vi "Filter_LDA.vi"(8 "Cluster in":T1={"Colour"=0, "Inst type"=enum."Pitot-static tube", "Inst name"="Manometer voltage", "Symbol"="U", "Code name"="", "Extra Info"="U", "Inst Array"=enum."PWA", "Extra Titles"=[], "Extra Values"=[], "Eng Values"=[], "Time (ms)"=[], "Voltage"=[], "U"=0.0, "u^2"=0.0, "u^3"=0.0, "u^4"=0.0, "Skew_u"=0.0, "Kurt_u"=0.0, "Sd Error in Mean"=0.0, "% u'/U"=0.0, "X"=0.0, "Y"=0.0, "Z"=0.0, "Spectra"={"First Name"="", "Second Name"="", "X axis name"="", "Y axis name"="", "X array"=[], "Y array"=[]}, "Autocorrelation"={"First Name"="", "Second Name"="", "X axis name"="", "Y axis name"="", "X array"=[], "Y array"=[]}, "Timescale integral to 25%"=0.0, "Sd Error in Variance"=0.0, "Calib File"=path "", "Calib Constants"=[], "Histogram"={"First Name"="", "Second Name"="", "X axis name"="", "Y axis name"="", "X array"=[], "Y array"=[]}, "Output Position"=FALSE, "Full Stats"=FALSE, "Weighting"=[], "Av Sampling Rate"=0.0, "Av No of Samples"=0.0, "Total Meas Time (s)"=0.0} {"Sd Error in Variance" format="%.2f"; "Skew_u" format="%.2f"; "% u'/U" format="%.2f"; "Sd Error in Mean" format="%.2f"; "Kurt_u" format="%.2f"; "u^4" format="%.2f"; "u^3" format="%.2f"; "U" format="%.2f"; "u^2" format="%.2f"}) -> (3 "Cluster Out":T1={"Colour"=0, "Inst type"=enum."Pitot-static tube", "Inst name"="Manometer voltage", "Symbol"="U", "Code name"="", "Extra Info"="U", "Inst Array"=enum."PWA", "Extra Titles"=[], "Extra Values"=[], "Eng Values"=[], "Time (ms)"=[], "Voltage"=[], "U"=0.0, "u^2"=0.0, "u^3"=0.0, "u^4"=0.0, "Skew_u"=0.0, "Kurt_u"=0.0, "Sd Error in Mean"=0.0, "% u'/U"=0.0, "X"=0.0, "Y"=0.0, "Z"=0.0, "Spectra"={"First Name"="", "Second Name"="", "X axis name"="", "Y axis name"="", "X array"=[], "Y array"=[]}, "Autocorrelation"={"First Name"="", "Second Name"="", "X axis name"="", "Y axis name"="", "X array"=[], "Y array"=[]}, "Timescale integral to 25%"=0.0, "Sd Error in Variance"=0.0, "Calib File"=path "", "Calib Constants"=[], "Histogram"={"First Name"="", "Second Name"="", "X axis name"="", "Y axis name"="", "X array"=[], "Y array"=[]}, "Output Position"=FALSE, "Full Stats"=FALSE, "Weighting"=[], "Av Sampling Rate"=0.0, "Av No of Samples"=0.0, "Total Meas Time (s)"=0.0} {"Sd Error in Variance" format="%.2f"; "Skew_u" format="%.2f"; "% u'/U" format="%.2f"; "Sd Error in Mean" format="%.2f"; "Kurt_u" format="%.2f"; "u^4" format="%.2f"; "u^3" format="%.2f"; "U" format="%.2f"; "u^2" format="%.2f"})   [LabVIEW 2011]
uses:
  Controls/Analysis_info_cluster.ctl
  Controls/Inst_type.ctl
  Controls/Instrument_Array.ctl
  Controls/XY_Plot_Cluster.ctl
  <vilib>/gmath/NI_Gmath.lvlib
panel:
  in  "Cutoff frequency (Hz)":dbl=25.0
  out "Numeric":dbl
  in  "method":i32(ring) items=["nearest", "linear", "spline", "cubic Hermite", "Lagrange"]
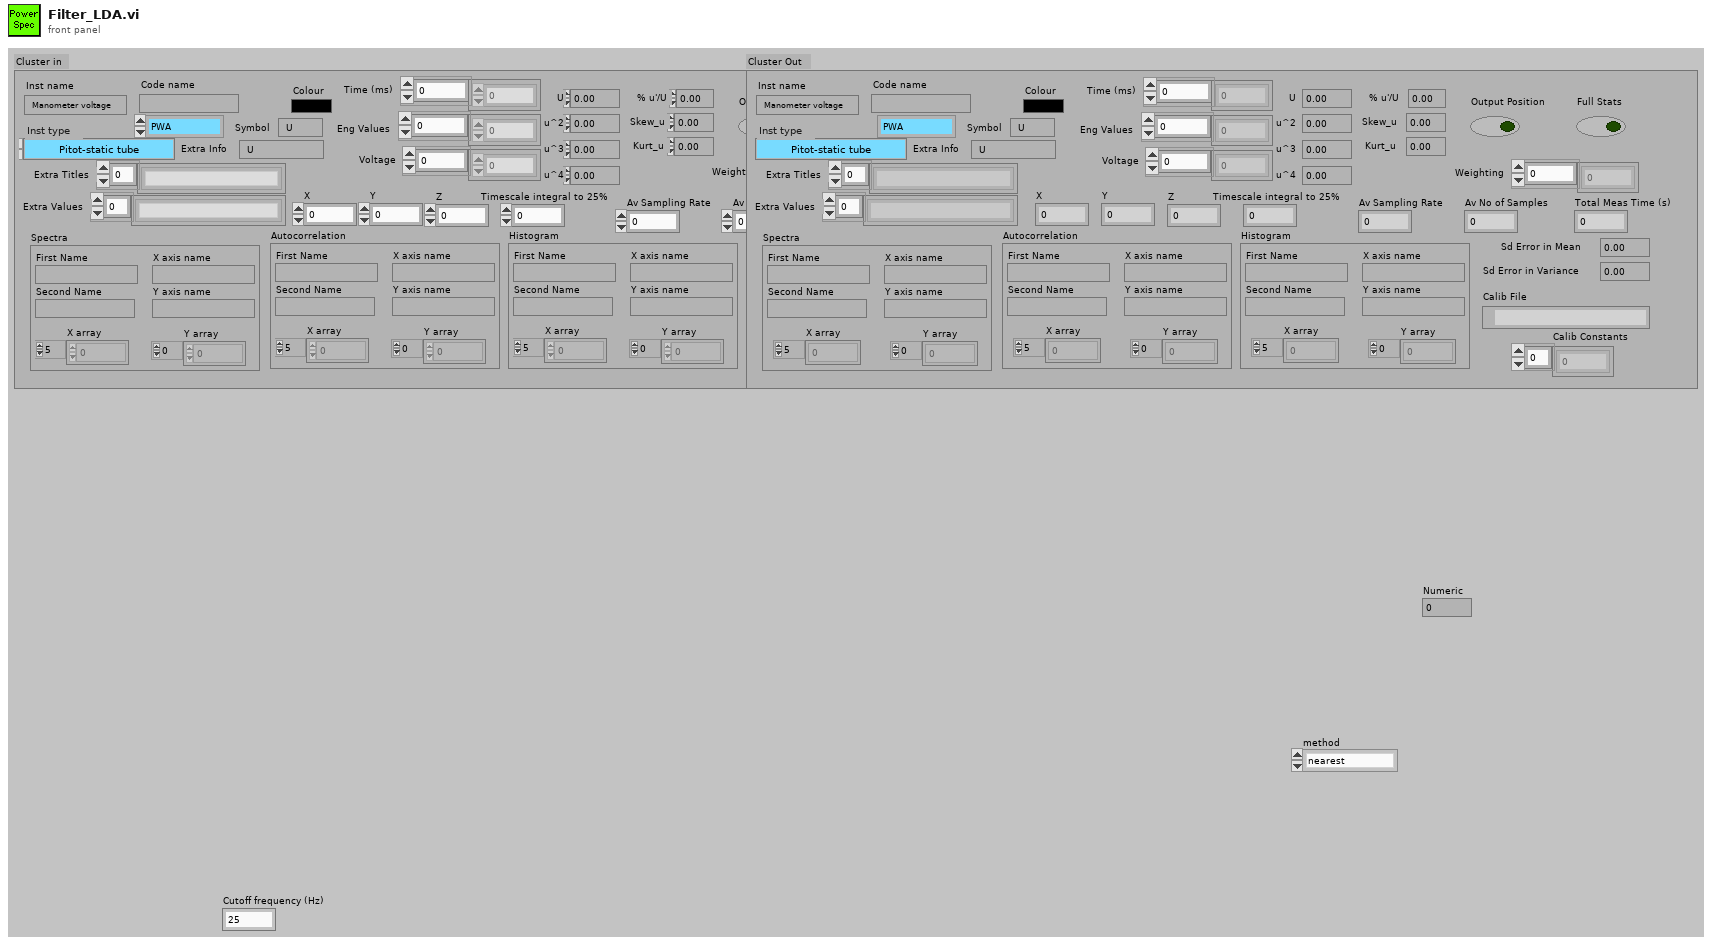
[diagram p1: front panel]
types:
  T1 = typedef "Analysis_info_cluster.ctl" = cluster{"Colour":u32, "Inst type":T2, "Inst name":string, "Symbol":string, "Code name":string, "Extra Info":string, "Inst Array":T3, "Extra Titles":string[], "Extra Values":string[], "Eng Values":dbl[], "Time (ms)":dbl[], "Voltage":dbl[], "U":dbl, "u^2":dbl, "u^3":dbl, "u^4":dbl, "Skew_u":dbl, "Kurt_u":dbl, "Sd Error in Mean":dbl, "% u'/U":dbl, "X":dbl, "Y":dbl, "Z":dbl, "Spectra":T4, "Autocorrelation":T4, "Timescale integral to 25%":dbl, "Sd Error in Variance":dbl, "Calib File":path, "Calib Constants":dbl[], "Histogram":T4, "Output Position":bool, "Full Stats":bool, "Weighting":dbl[], "Av Sampling Rate":dbl, "Av No of Samples":dbl, "Total Meas Time (s)":dbl}
  T2 = typedef "Inst_type.ctl" = enum16{"Propeller anemometer", "Raw voltage", "Pressure Transducer", "Pitot-static tube", "Preston tube", "Hot wire", "Cross wire 1", "Cross wire 2", "Generic Linear", "Generic Polynomial", "Generic BackPoly", "Fast FID", "Thermocouple", "Cold wire", "Pulsed Wire", "LDA Vel", "LDA Tran time", "LDA Arr time"}
  T3 = typedef "Instrument_Array.ctl" = enum16{"PWA", "LDA", "Analogue"}
  T4 = typedef "XY_Plot_Cluster.ctl" = cluster{"First Name":string, "Second Name":string, "X axis name":string, "Y axis name":string, "X array":dbl[], "Y array":dbl[]}
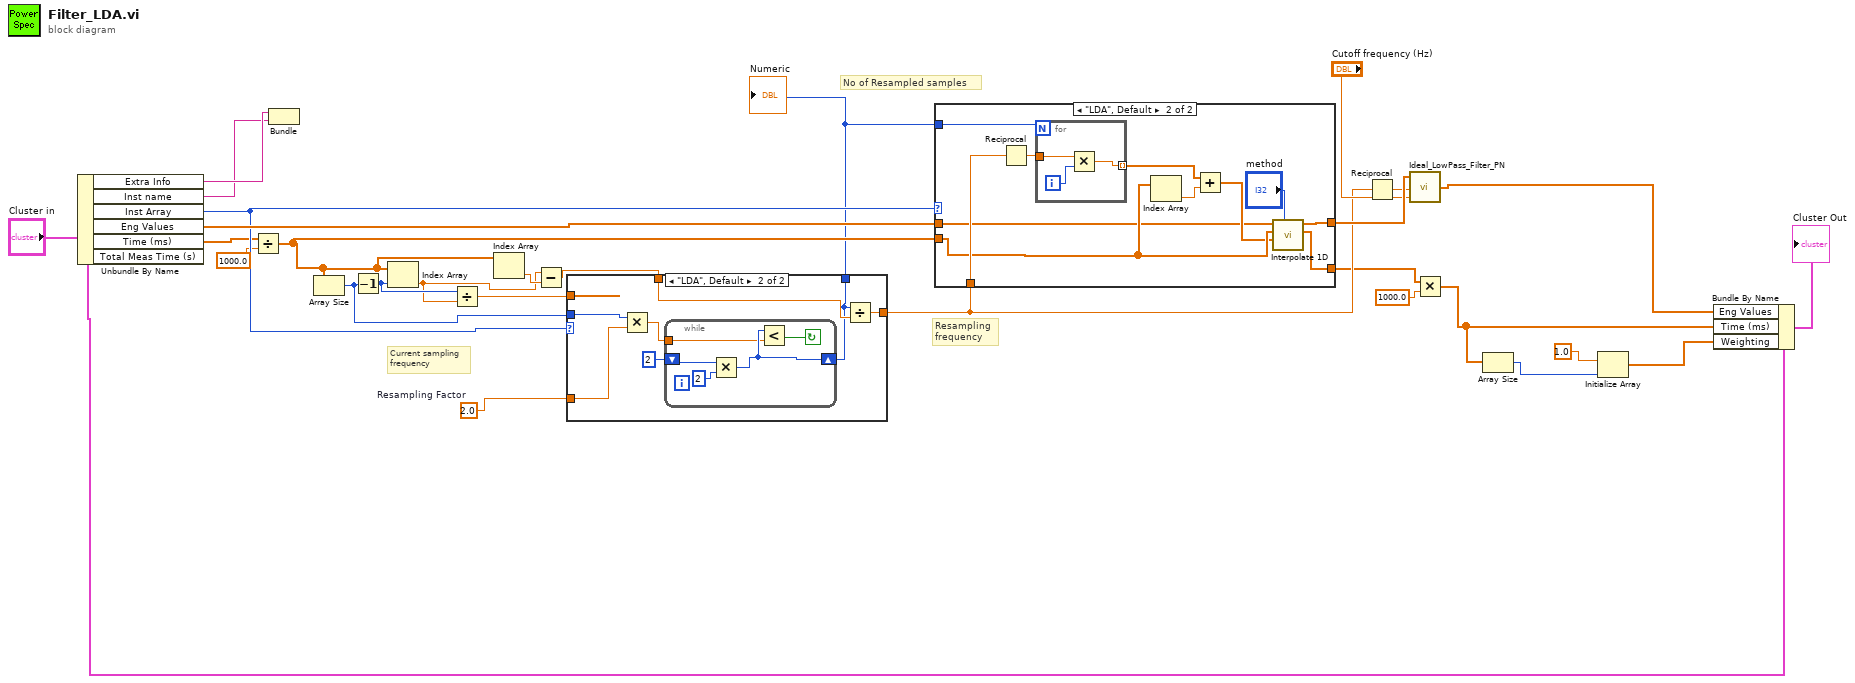
[diagram p0: block diagram]
diagram:
  w7 = 2.0  # Resampling Factor
  # "Current sampling\nfrequency"
  # "No of Resampled samples"
  # "Resampling\nfrequency"
  n1 = Unbundle By Name("Cluster in") -> ("Extra Info"=w23:string, "Inst name"=w22:string, "Inst Array"=w27:T3, "Eng Values"=w28:dbl[], "Time (ms)"=w25:dbl[])  [unwired: 1 out]
  n2 = Divide(x=w25, y=1000.0) -> (x/y=w24:dbl[])
  n3 = Bundle("Extra Info"=w23, "Inst name"=w22) -> ()  [unwired: 1 in, 1 out]
  n4 = Array Size(array=w24) -> (size(s)=w8:i32)
  n5 = Decrement(x=w8) -> (x-1=w9:i32)
  n6 = Index Array(array=w24, index=w9) -> (element=w4:dbl)
  n7 = Divide(x=w9, y=w4) -> (x/y=w10:dbl)
  n8 = Index Array(array=w24) -> (element=w6:dbl)  [unwired: 1 in]
  n9 = Subtract(x=w4, y=w6) -> (x-y=w5:dbl)
  n10 = case shown="\"LDA\", Default" w27 {
    tunnel: w10 -> [w30 _]
    tunnel: w5 -> [_ w37]
    tunnel: [w30 w36] -> w15
    tunnel: w8 -> [w29 w34]
    tunnel: [w29 w33] -> w21
    tunnel: w7 -> [_ w32]
    frame "Analogue" {
    }
    frame "LDA", Default {
      n11 = Multiply(x=w34, y=w32) -> (x*y=w35:dbl)
      n12 = while {
        shift-right: [w40] -> w33
        shift-left: 2 -> [w42]
        tunnel: w35 -> [w38]
        stop <- w39 continue-if-true
        n13 = Multiply(x=w42, y=2) -> (x*y=w40:i32)
        n14 = Less?(x=w40, y=w38) -> (x < y?=w39:bool)
      }
      n15 = Divide(x=w33, y=w37) -> (x/y=w36:dbl)
    }
  }
  "Numeric" <- w21
  n16 = case shown="\"LDA\", Default" w27 {
    tunnel: w28 -> [w44 w46]
    tunnel: w24 -> [w43 w50]
    tunnel: [w44 w54] -> w18
    tunnel: w21 -> [_ w53]
    tunnel: w15 -> [_ w51]
    tunnel: [w43 w45] -> w2
    frame "Analogue" {
    }
    frame "LDA", Default {
      n17 = Reciprocal(x=w51) -> (1/x=w52:dbl)
      n18 = for {
        N: w53 -> [_]
        tunnel: w52 -> [w58]
        tunnel: [w56] -> w48 mode=indexing
        i -> [w57]
        n19 = Multiply(x=w58, y=w57) -> (x*y=w56:dbl)
      }
      n20 = Index Array(array=w50) -> (element=w49:dbl)  [unwired: 1 in]
      n21 = Add(x=w48, y=w49) -> (x+y=w47:dbl[])
      n22 = call <vilib>:"Interpolate 1D.vi"("method"="method", "xi"=w47, "X"=w50, "Y"=w46) -> ("xi used"=w45:dbl[], "yi"=w54:dbl[])  [unwired: 2 in, 4 out]
    }
  }
  n23 = Reciprocal(x=w15) -> (1/x=w16:dbl)
  n24 = call "Ideal_LowPass_Filter_PN.vi"("Cutoff frequency (Hz)"="Cutoff frequency (Hz)", "dt (s)"=w16, "1D Data (uniform spacing)"=w18) -> ("Low-pass filtered 1D Data"=w14:dbl[])
  n25 = Multiply(x=w2, y=1000.0) -> (x*y=w1:dbl[])
  n26 = Array Size(array=w1) -> (size(s)=w13:i32)
  n27 = Initialize Array(1.0, w13) -> (w11:dbl[])
  n28 = Bundle By Name(cluster="Cluster in", "Eng Values"=w14, "Time (ms)"=w1, "Weighting"=w11) -> (→"Cluster Out":T1)
